vi "参数配置.vi"(8 "error in (no error)":errorcluster, 11 "配置":T1={"编码器工程变换系数_计数值"=0.0, "编码器工程变换系数_工程值"=0.0, "最小精度设置"=0.01, "剖面校正值设定"=0.0, "软限位最大值"=25.0, "软限位最小值"=2.0, "剖面待机位置设定"=0.0} {"剖面待机位置设定" format="%#_6f m"; "软限位最小值" format="%#_6f m"; "软限位最大值" format="%#_6f m"; "剖面校正值设定" format="%#_6f m"; "最小精度设置" format="%#.6f"; "编码器工程变换系数_工程值" format="%#_6f m"; "编码器工程变换系数_计数值" format="%#_6f ps"}) -> (0 "error out":errorcluster)   [LabVIEW 2016, in "PLC.lvlib"]
uses:
  PLC.lvlib
  <vilib>/Plasmionique/MB Master/MB_Master_Serial/MB_Master_Serial.lvclass
  C:/Program Files (x86)/National Instruments/LabVIEW 2016/vi.lib/Plasmionique/MB Master/MB_Master/MB_Master.lvclass
  <vilib>/Plasmionique/MB Master/MB Master.lvlib
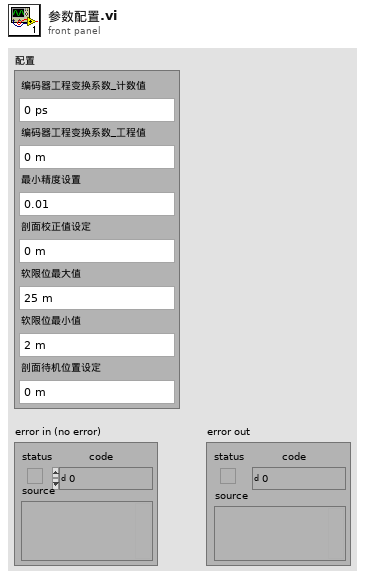
[diagram p1: front panel]
types:
  T1 = cluster{"编码器工程变换系数_计数值":sgl, "编码器工程变换系数_工程值":sgl, "最小精度设置":sgl, "剖面校正值设定":sgl, "软限位最大值":sgl, "软限位最小值":sgl, "剖面待机位置设定":sgl}
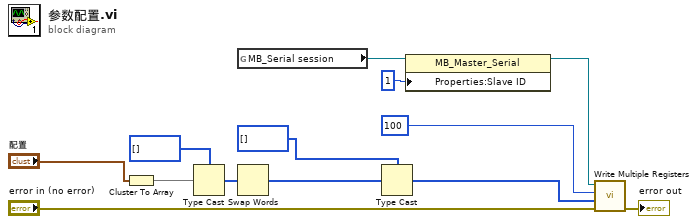
[diagram p0: block diagram]
diagram:
  n1 = Cluster To Array(cluster="配置") -> (array=w9:sgl[])
  n2 = Type Cast(type=u32[] [], x=w9) -> (*(type *) &x=w7:u32[])
  n3 = global read "中间变量.vi" "MB_Serial session"() -> (w3:refnum<class "MB_Master_Serial.lvclass">)
  n4 = Swap Words(1:w7) -> (0:w6:u32[])
  n5 = Type Cast(type=u16[] [], x=w6) -> (*(type *) &x=w4:u16[])
  n6 = property class="MB_Master_Serial"(reference=w3, "Properties:Slave ID"=u8 1 ("Slave ID")) -> (reference out=w2:refnum<class "MB_Master_Serial.lvclass">)  [unwired: 1 in, 1 out]
  n7 = call <vilib>:"Write Multiple Registers.vi"("error in (no error)"="error in (no error)", "values"=w4, "starting address"=u16 100, "MB session in"=w2) -> ("error out"=→"error out":errorcluster)  [unwired: 6 in, 1 out]
